vi "Done.vi"(8 "error in (no error)":errorcluster, 11 "Terminal Timeout in":refnum<class "Terminal Timeout.lvclass">) -> (0 "error out":errorcluster, 3 "Terminal Timeout out":refnum<class "Terminal Timeout.lvclass">)   [LabVIEW 2016, in "CLD Exam - ATM.lvlib" / "Terminal Timeout.lvclass"]
uses:
  Terminal Timeout.lvclass
  Mediator/Classes/Mediated Synchronous Actor/Mediated Synchronous Actor.lvclass
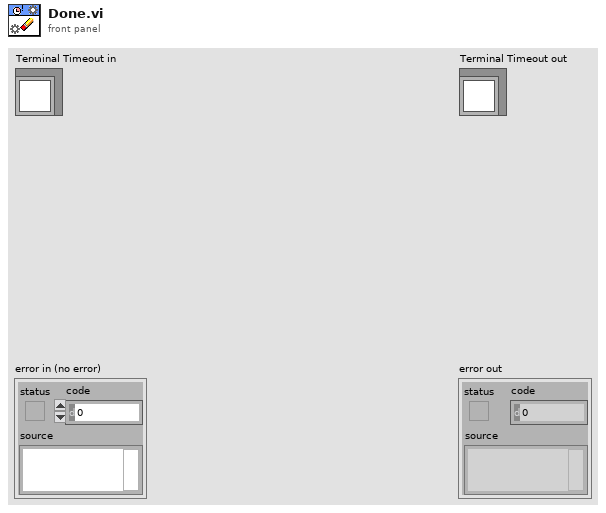
[diagram p1: front panel]
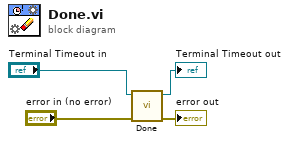
[diagram p0: block diagram]
diagram:
  n1 = call-parent "Done.vi"("error in (no error)"="error in (no error)", "Mediated Synchronous Actor in"="Terminal Timeout in") -> ("error out"=→"error out":errorcluster, "Mediated Synchronous Actor out"=→"Terminal Timeout out":refnum<class "Terminal Timeout.lvclass">)  [unwired: 8 in]
